vi "REWORK_LOGIN_scan_barcode.vi"(8 "error_in":errorcluster, 11 "all_config_info":T1={"main_ini_file"={"SQL Driver"="", "SQL Server"="", "SQL Database"="", "SQL UID"="", "User table"="", "default language"="", "SCANNER COM port"=0, "SCANNER Baud rate"=0, "SCANNER Data bits"=0, "SCANNER Pairity"=enum."None", "SCANNER Stop bits"=10, "SCANNER Flow control"=0, "SCANNER Termination char"=0, "ST 140 name"="", "ST 140 listener IP"="", "ST 140 listener port"=0, "logout timeout [ms]"=0}, "SQL Password"="", "queue_refnums"={"MAIN_queue"=refnum, "SCANNER_queue"=refnum, "SCANNER_data"=refnum}} {"main_ini_file"."SCANNER Flow control" items=["None"=0, "XON/XOFF"=1, "RTS/CTS"=2, "DTR/DSR"=4]; "main_ini_file"."SCANNER Stop bits" items=["1.0"=10, "1.5"=15, "2.0"=20]}) -> (0 "error_out":errorcluster, 2 "Canceled?":bool, 3 "barcode":string)   [LabVIEW 2019]
uses:
  ini/typedef/REWORK_all_config_info.ctl
  ini/typedef/REWORK_main_ini_file.ctl
  queues/typedef/REWORK_queue_refnums.ctl
  queues/typedef/REWORK_MAIN_queue_element.ctl
  REWORK_MAIN_sequence_state.ctl
  queues/typedef/REWORK_SCANNER_queue_element.ctl
  SCANNER/REWORK_SCANNER_sequence_state.ctl
  _misc/AULocalize/SubVIs/RegisterVI.vi
panel:
  out "waiting_for_barcode_scan_msg":string caption="(ий)Waiting for barcode scan..."
  in  "cancel_barcode_scan":bool
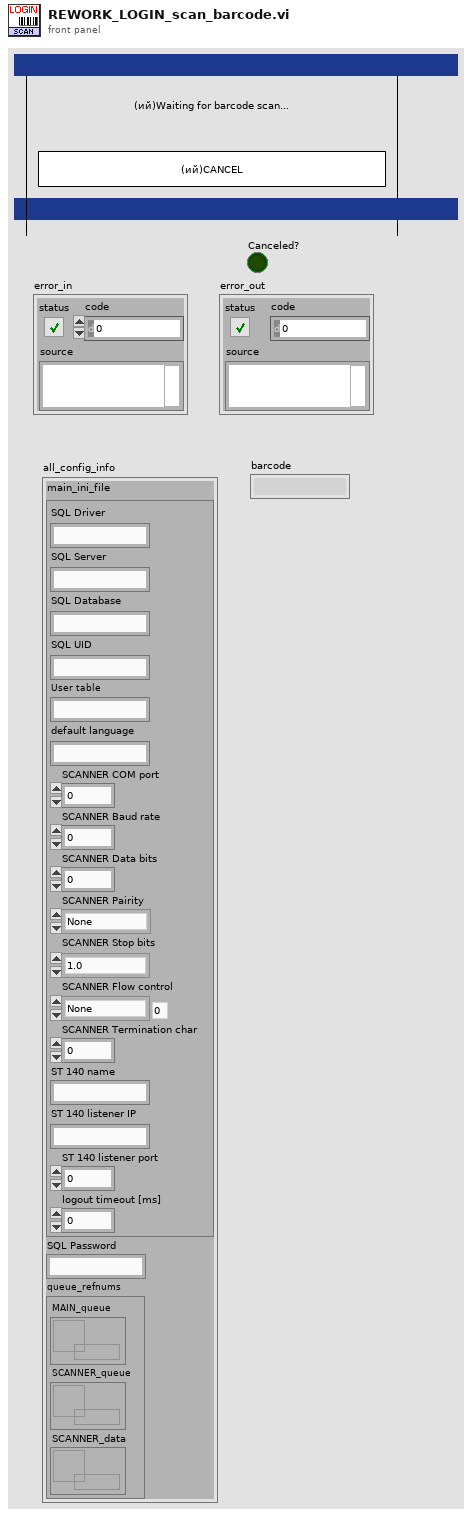
[diagram p1: front panel]
types:
  T1 = typedef "REWORK_all_config_info.ctl" = cluster{"main_ini_file":T2, "SQL Password":string, "queue_refnums":T3}
  T2 = typedef "REWORK_main_ini_file.ctl" = cluster{"SQL Driver":string, "SQL Server":string, "SQL Database":string, "SQL UID":string, "User table":string, "default language":string, "SCANNER COM port":u16, "SCANNER Baud rate":u32, "SCANNER Data bits":u16, "SCANNER Pairity":enum16{"None", "Odd", "Even", "Mark", "Space"}, "SCANNER Stop bits":u16, "SCANNER Flow control":u16, "SCANNER Termination char":u8, "ST 140 name":string, "ST 140 listener IP":string, "ST 140 listener port":u16, "logout timeout [ms]":i32}
  T3 = typedef "REWORK_queue_refnums.ctl" = cluster{"MAIN_queue":refnum<queue>, "SCANNER_queue":refnum<queue>, "SCANNER_data":refnum<queue>}
  T4 = typedef "REWORK_SCANNER_queue_element.ctl" = cluster{"state":T5, "variable":variant}
  T5 = typedef "REWORK_SCANNER_sequence_state.ctl" = enum16{"initialize", "get_next_state", "read", "cancel_read", "error", "stop"}
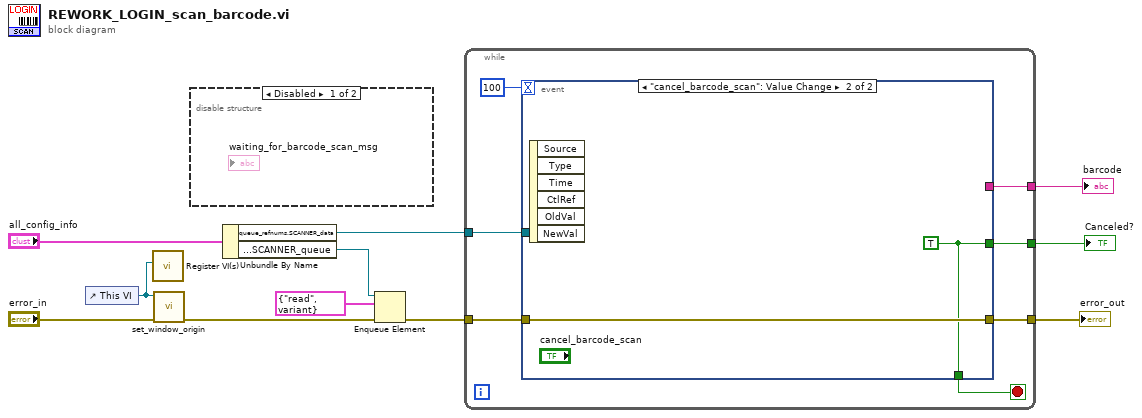
[diagram p0: block diagram]
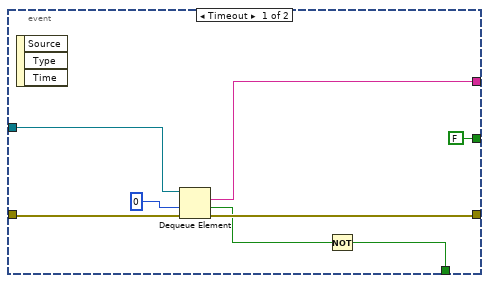
[diagram p3: hidden frame]
diagram:
  n1 = control-ref of="This VI"() -> (w1:refnum<vi>)
  n2 = call-poly "Register VI(s).vi"("VI Ref"=w1) -> ()  [unwired: 9 in, 2 out]
  n3 = call "set_window_origin.vi"("error_in"="error_in", "this_vi_reference"=w1) -> ("error_out"=w6:errorcluster)  [unwired: 9 in]
  n4 = disable-structure shown="Disabled" {
    frame Disabled {
    }
    frame Enabled {
    }
  }
  n5 = Unbundle By Name("all_config_info") -> ("queue_refnums.SCANNER_data"=w8:refnum<queue>, "queue_refnums.SCANNER_queue"=w4:refnum<queue>)
  n6 = Enqueue Element(queue=w4, element=T4 {"state"=enum."read", "variable"=variant}, error in (no error)=w6) -> (error out=w5:errorcluster)  [unwired: 1 in, 2 out]
  n7 = while {
    tunnel: w5 -> [w18]
    tunnel: [w17] -> w11
    tunnel: w8 -> [w14]
    tunnel: [w13] -> w7
    tunnel: [w12] -> w2
    stop <- w15 stop-if-true
    n8 = event shown="[1] \"cancel_barcode_scan\": Value Change" {
      selector: _ -> [_ _]
      dyn-events: _ -> [_ _]
      timeout: 100 -> [_ _]
      tunnel: w18 -> [w25 w28]
      tunnel: [w24 w28] -> w17
      tunnel: [w20 w27] -> w15
      tunnel: w14 -> [w26 _]
      tunnel: [w21 _] -> w13
      tunnel: [FALSE w27] -> w12
      event Timeout {
        n9 = event-data() -> ()  [unwired: 1 in, 3 out]
        n10 = Dequeue Element(queue=w26, timeout in ms (-1)=0, error in (no error)=w25) -> (element=w21:string, timed out?=w22:bool, error out=w24:errorcluster)  [unwired: 1 out]
        n11 = Not(x=w22) -> (.not. x?=w20:bool)
      }
      event "cancel_barcode_scan": Value Change {
        w27 = TRUE
        n12 = event-data() -> ()  [unwired: 1 in, 6 out]
      }
    }
  }
  "error_out" <- w11
  "barcode" <- w7
  "Canceled?" <- w2
